vi "MHM Initialize.vi"(8 "error in (no error)":errorcluster, 11 "ulMHMHandle":u32) -> (0 "error out":errorcluster, 3 "function return":u32)   [LabVIEW 2017, in "MHM_1SL_interface.lvlib"]
uses:
  MHM_1SL_interface.lvlib
  lib/MHM_1SL_interface.dll
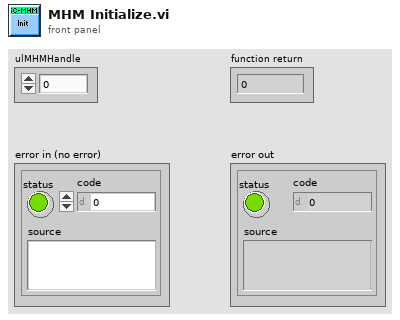
[diagram p1: front panel]
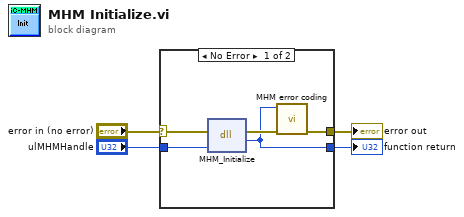
[diagram p0: block diagram]
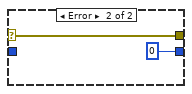
[diagram p2: hidden frame]
diagram:
  n1 = case shown="No Error" "error in (no error)" {
    selector: "error in (no error)" -> [w9 w11]
    tunnel: "ulMHMHandle" -> [w8 _]
    tunnel: [w6 w11] -> w2
    tunnel: [w5 u32 0 ("return type")] -> w1
    frame No Error {
      n2 = dll-call lib="C:/workspace/project/scancon/sw/SSI_Tool/DUT_Interface/lv_interface/lib/MHM_1SL_interface.dll" fn="MHM_Initialize"(error in=w9, "ulMHMHandle"=w8) -> (error out=w7:errorcluster, "return type"=w5:u32)  [unwired: 3 in, 1 out]
      n3 = call "MHM error coding.vi"("error in (no error)"=w7, "function return in"=w5) -> ("error out"=w6:errorcluster)  [unwired: 9 in]
    }
    frame Error {
    }
  }
  "function return" <- w1
  "error out" <- w2
